vi "Main.vi"() -> ()   [LabVIEW 2024]
doc: "This Continuous Measurement sample project is based on the Queued Message Handler template.\n\nThe Event Handling Loop generates messages based on user interface actions.\n\nThe Message Handling Loop processes messages generated by the Event Handling Loop, or by other messages. There are also Acquisition and Logging message handling loop subVIs, and a chart updating loop."
uses:
  Acquisition/Acquisition.lvlib
  Logging/Logging.lvlib
  support/User Event - Stop/User Event - Stop.lvlib
  controls/UI Data.ctl
  support/Message Queue/Message Queue.lvlib
  support/Message Queue/Enqueue Message (Single).vi
  <vilib>/ErrorRing/Error Ring.xnode
  controls/UI State.ctl
  <vilib>/Utility/error.llb/Error Cluster From Error Code.vi
  controls/channelDefinition.ctl
  controls/self.ctl
  controls/dataRefs.ctl
panel:
  out "Data":dbl[][](graph)
  in  "Force Trigger":bool
  in  "Start":bool
  in  "Stop":bool
  out "Status":string
  in  "Exit":bool
  # "Continuous Measurement and Logging (NI-DAQmx)"
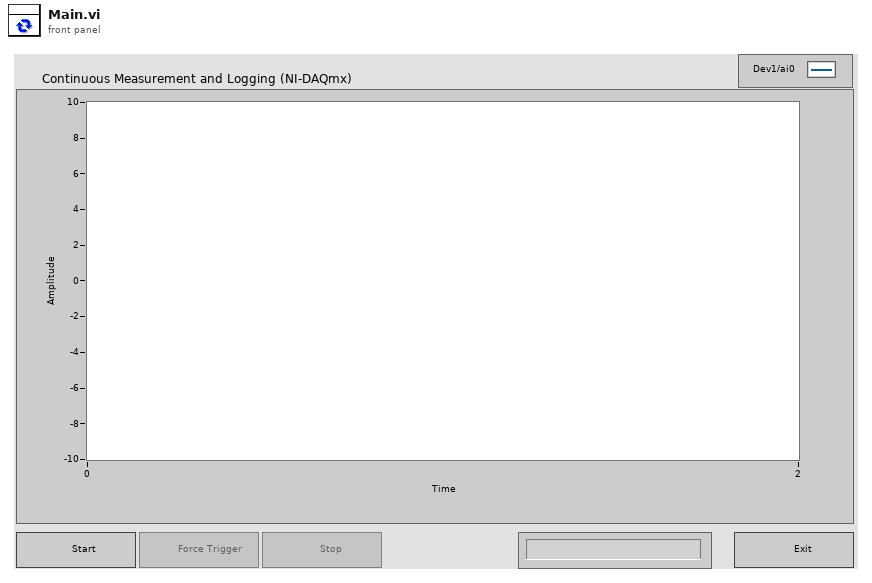
[diagram p1: front panel]
types:
  T1 = typedef "dataRefs.ctl" = cluster{"dataTypeConstant":cluster{"data":dbl[][], "refDes":string[]}, "user_I":refnum<notifier>, "user_O":refnum<notifier>, "daq_O":refnum<notifier>, "logging":refnum<queue>, "daq_I":refnum<queue>}
  T2 = typedef "self.ctl" = cluster{"refDes":string, "IP":string, "DI":i32, "DO":i32, "AI":i32, "AO":i32, "Description":string, "TC":i32, "channelDefinitions":T3[]}
  T3 = typedef "channelDefinition.ctl" = cluster{"channel":string, "refDes":string, "units":string, "slope":dbl, "offset":dbl, "type":string}
  T4 = typedef "UI State.ctl" = enum16{"Idle", "Acquiring and Logging", "Waiting for Exit", "Waiting for Exit (Acq Stopped)", "Waiting for Exit (Log Stopped)", "Waiting for Stop", "Waiting for Stop (Acq Stopped)", "Waiting for Stop (Log Stopped)"}
  T5 = typedef "UI Data.ctl" = cluster{"Start Ref":refnum<vi>, "Trigger Ref":refnum<vi>, "Stop Ref":refnum<vi>, "Settings Ref":refnum<vi>, "Status Ref":refnum<vi>, "Exit Ref":refnum<vi>, "Data Ref":refnum<vi>}
  T6 = typedef "Message Queue.lvlib/All Message Queues.ctl" = cluster{"UI":refnum<queue>, "Acquisition":refnum<queue>, "Logging":refnum<queue>}
  T7 = enum8{"Enabled", "Disabled", "Disabled and Grayed Out"}
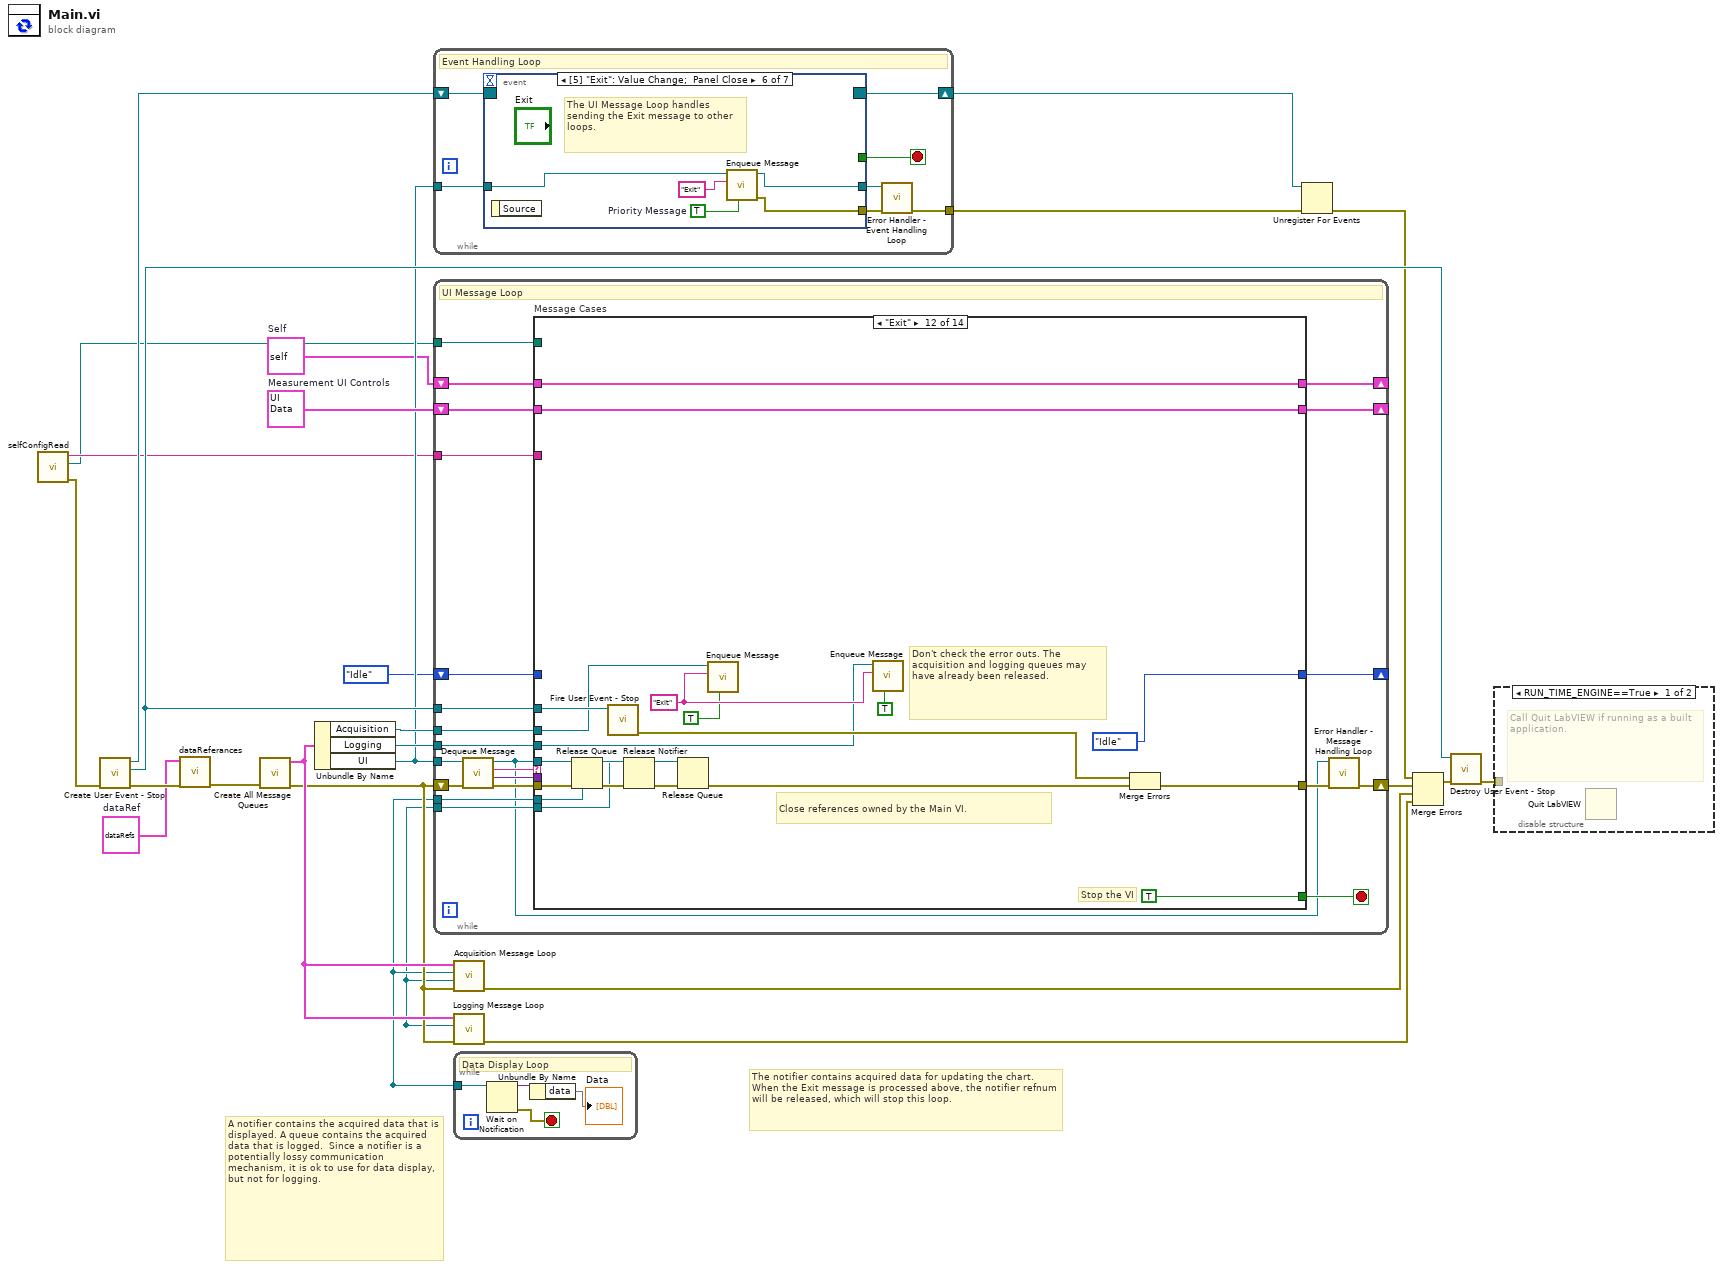
[diagram p0: block diagram]
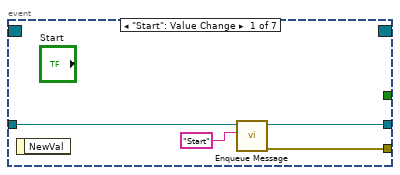
[diagram p3: hidden frame]
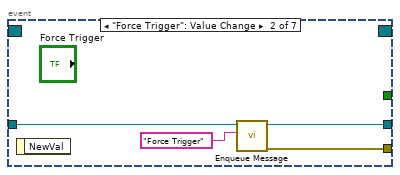
[diagram p4: hidden frame]
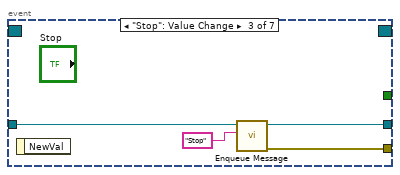
[diagram p5: hidden frame]
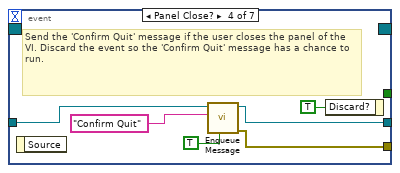
[diagram p6: hidden frame]
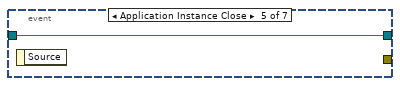
[diagram p7: hidden frame]
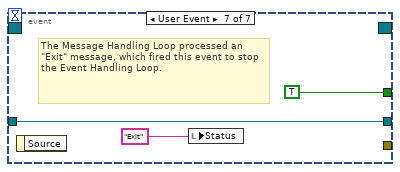
[diagram p8: hidden frame]
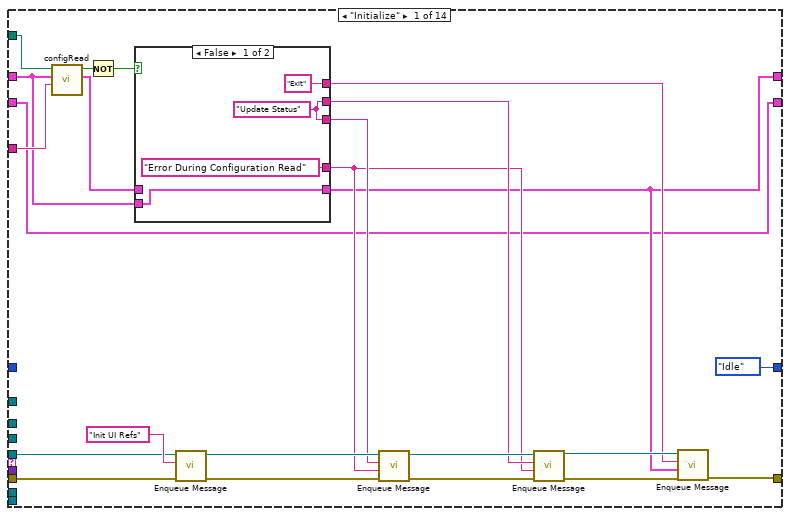
[diagram p9: hidden frame]
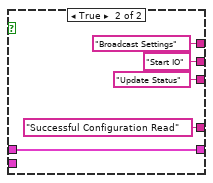
[diagram p10: hidden frame]
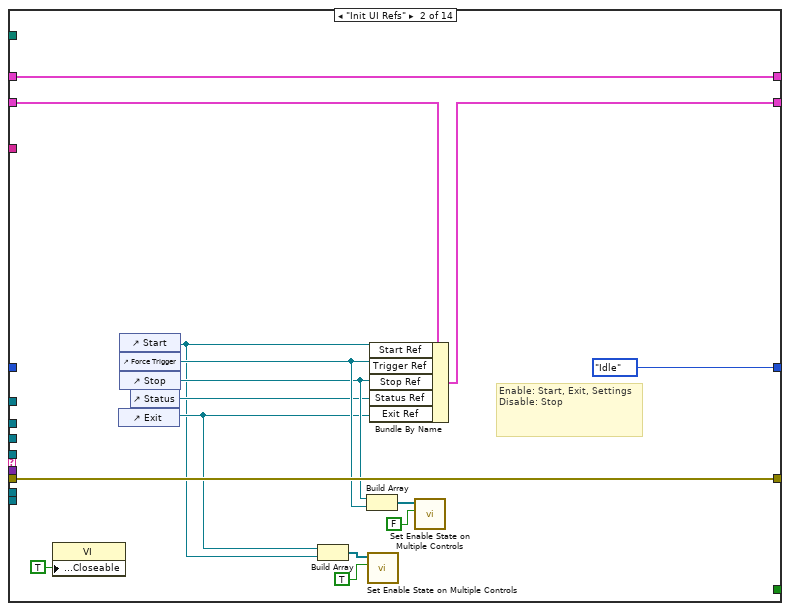
[diagram p11: hidden frame]
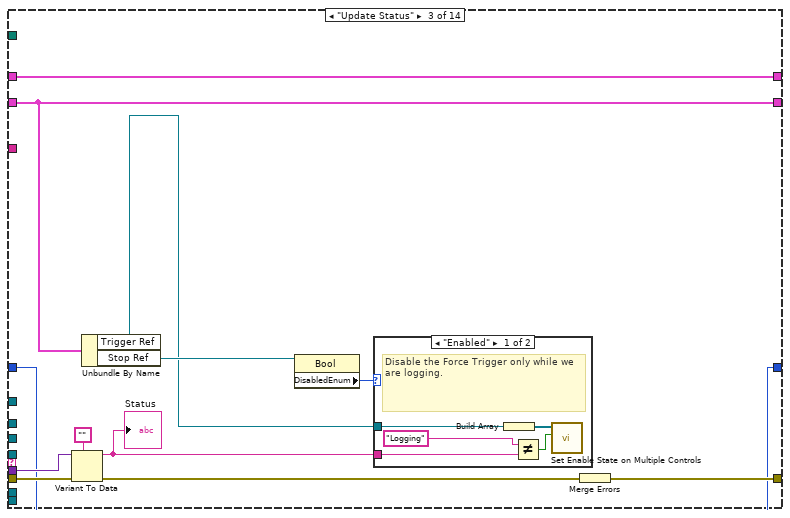
[diagram p12: hidden frame]
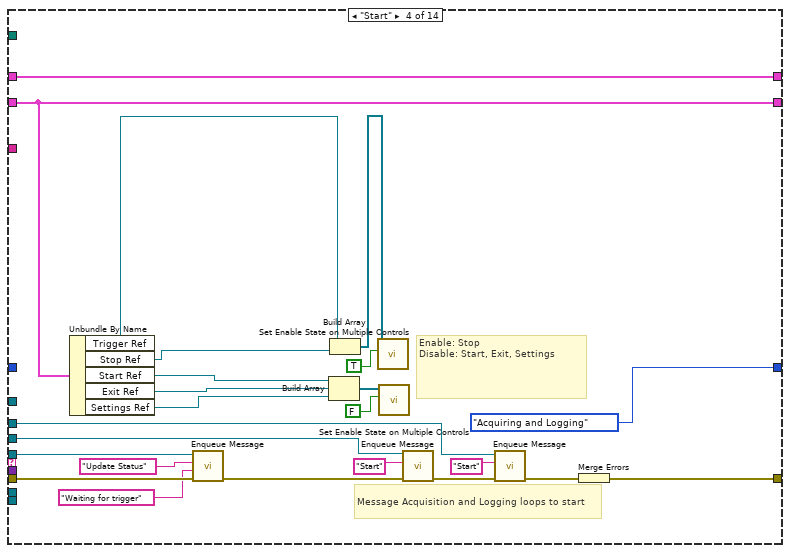
[diagram p14: hidden frame]
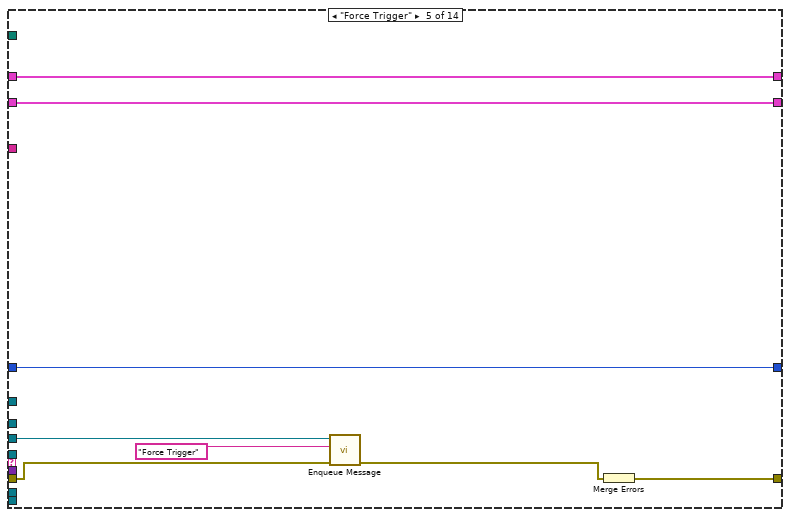
[diagram p15: hidden frame]
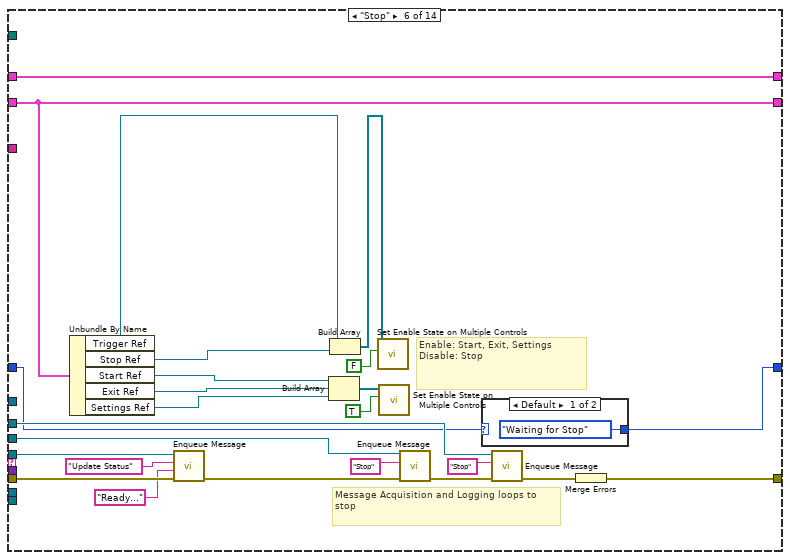
[diagram p16: hidden frame]
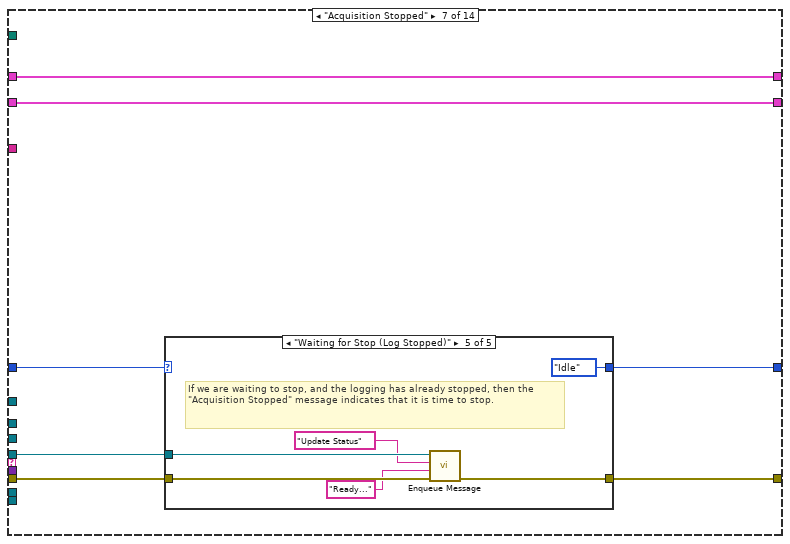
[diagram p18: hidden frame]
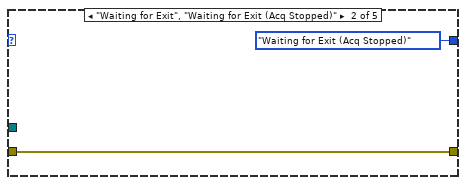
[diagram p20: hidden frame]
diagram:
  w1 = T1 {"dataTypeConstant"={"data"=[], "refDes"=[]}, "user_I"=refnum, "user_O"=refnum, "daq_O"=refnum, "logging"=refnum, "daq_I"=refnum}  # dataRef
  w9 = T2 {"refDes"="ERR000", "IP"="localhost", "DI"=0, "DO"=0, "AI"=0, "AO"=0, "Description"="ERR", "TC"=0, "channelDefinitions"=[]}  # Self
  w15 = T5 {"Start Ref"=refnum, "Trigger Ref"=refnum, "Stop Ref"=refnum, "Settings Ref"=refnum, "Status Ref"=refnum, "Exit Ref"=refnum, "Data Ref"=refnum}  # Measurement UI Controls
  # "A notifier contains the acquired data that is displayed. A queue contains the acquired data that is logged.  Since a notifier is a potentially lossy communication mechanism, it is ok to use for data display, but not for logging."
  # "The notifier contains acquired data for updating the chart. When the Exit message is processed above, the notifier refnum will be released, which will stop this loop."
  n1 = call "selfConfigRead.vi"() -> ("error out"=w7:errorcluster, "configPath"=w6:path, "refDes"=w8:string)  [unwired: 9 in]
  n2 = call "Create User Event - Stop.vi"("error in (no error)"=w7) -> ("error out"=w3:errorcluster, "User Event - Stop"=w22:refnum<user-event>, "Stop Event Registration Refnum"=w23:refnum<event-registration>)  [unwired: 8 in]
  n3 = call "dataReferances.vi"("error in (no error)"=w3, "dataRefIn"=w1) -> ("error out"=w2:errorcluster)  [unwired: 8 in, 1 out]
  n4 = call "Create All Message Queues.vi"("error in (no error)"=w2) -> ("error out"=w18:errorcluster, "Message Queues out"=w20:T6)  [unwired: 9 in]
  n5 = Unbundle By Name(w20) -> ("Acquisition"=w14:refnum<queue>, "Logging"=w13:refnum<queue>, "UI"=w12:refnum<queue>)
  n6 = while {
    tunnel: w12 -> [w32]
    tunnel: [w27] -> w25
    shift-right: [w31] -> w16
    shift-left: w23 -> [w33]
    stop <- w30 stop-if-true
    # "Event Handling Loop"
    n7 = event shown="[5] \"Exit\": Value Change;  Panel Close" {
      selector: w33 -> [_ _ _ _ _ _ _]
      dyn-events: [_ _ _ _ _ _ _] -> w31
      timeout: _ -> [_ _ _ _ _ _ _]
      tunnel: [_ _ _ _ _ _ TRUE ("Discard?")] -> w30
      tunnel: w32 -> [w35 w40 w44 w51 w52 w54 w58]
      tunnel: [w37 w39 w43 w46 _ w57 _] -> w28
      tunnel: [w34 w38 w42 w47 w52 w53 w58] -> w29
      event "Start": Value Change {
        n8 = event-data() -> ()  [unwired: 1 in, 1 out]
        n9 = call-poly "Enqueue Message.vi"("Message"="Start", "Message Queue"=w35) -> ("error out"=w37:errorcluster, "dup Message Queue"=w34:refnum<queue>)  [unwired: 8 in]
      }
      event "Force Trigger": Value Change {
        n10 = event-data() -> ()  [unwired: 1 in, 1 out]
        n11 = call-poly "Enqueue Message.vi"("Message"="Force Trigger", "Message Queue"=w40) -> ("error out"=w39:errorcluster, "dup Message Queue"=w38:refnum<queue>)  [unwired: 8 in]
      }
      event "Stop": Value Change {
        n12 = event-data() -> ()  [unwired: 1 in, 1 out]
        n13 = call-poly "Enqueue Message.vi"("Message"="Stop", "Message Queue"=w44) -> ("error out"=w43:errorcluster, "dup Message Queue"=w42:refnum<queue>)  [unwired: 8 in]
      }
      event Panel Close? {
        # "Send the 'Confirm Quit' message if the user closes the panel of the VI. Discard the event so the 'Confirm Quit' message has a chance to run."
        n14 = event-data() -> ()  [unwired: 1 in, 1 out]
        n15 = call-poly "Enqueue Message.vi"("Priority Message? (F)"=TRUE, "Message"="Confirm Quit", "Message Queue"=w51) -> ("error out"=w46:errorcluster, "dup Message Queue"=w47:refnum<queue>)  [unwired: 7 in]
        n16 = event-data("Discard?"=TRUE) -> ()  [unwired: 1 in, 1 out]
      }
      event Application Instance Close {
        n17 = event-data() -> ()  [unwired: 1 in, 1 out]
      }
      event "Exit": Value Change; Panel Close {
        w55 = TRUE  # Priority Message
        # "The UI Message Loop handles sending the Exit message to other loops."
        n18 = event-data() -> ()  [unwired: 1 in, 1 out]
        n19 = call-poly "Enqueue Message.vi"("Priority Message? (F)"=w55, "Message"="Exit", "Message Queue"=w54) -> ("error out"=w57:errorcluster, "dup Message Queue"=w53:refnum<queue>)  [unwired: 7 in]
      }
      event User Event {
        # "The Message Handling Loop processed an \"Exit\" message, which fired this event to stop the Event Handling Loop."
        n20 = event-data() -> ()  [unwired: 1 in, 1 out]
        n21 = local write "Status"("Exit" ("Exit String")) -> ()
      }
    }
    n22 = call "Error Handler - Event Handling Loop.vi"("error in (no error)"=w28, "Message Queue"=w29) -> ("dup error in"=w27:errorcluster)  [unwired: 8 in, 1 out]
  }
  n23 = Unregister For Events(event registration refnum=w16, error in=w25) -> (error out=w17:errorcluster)
  n24 = while {
    tunnel: w12 -> [w76]
    tunnel: w22 -> [w81]
    shift-right: [w66] -> w26
    shift-left: w18 -> [w80]
    shift-right: [w75] -> _
    shift-left: w9 -> [w74]
    shift-right: [w72] -> _
    shift-left: w15 -> [w73]
    tunnel: w14 -> [w71]
    tunnel: w13 -> [w70]
    tunnel: [w69] -> w5
    tunnel: w4 -> [w68]
    shift-right: [w63] -> _
    shift-left: UI_State."Idle" ("UI State") -> [w64]
    tunnel: w6 -> [w62]
    tunnel: w8 -> [w61]
    stop <- w82 stop-if-true
    # "UI Message Loop"
    n25 = call "Dequeue Message.vi"("error in (no error)"=w80, "Message Queue"=w76) -> ("error out"=w79:errorcluster, "Message Data"=w77:variant, "Message"=w78:string, "dup Message Queue"=w65:refnum<queue>)  [unwired: 6 in]
    n26 = case "Message Cases" shown="\"Exit\"" w78 {
      selector: w78 -> [_ _ _ _ _ _ _ _ _ _ _ _ _ w332]
      tunnel: w65 -> [w104 _ _ w169 _ w202 w206 w231 _ w272 w282 w315 _ _]
      tunnel: w79 -> [w103 w129 w140 w168 w175 w201 w208 w233 w262 w276 w281 w323 w330 _]
      tunnel: [w98 w129 w141 w170 w178 w203 w207 w232 w265 w267 w280 w324 w329 w333] -> w67
      tunnel: [_ _ _ _ _ _ _ _ _ _ _ TRUE _ _] -> w82
      tunnel: w77 -> [_ _ w139 _ _ _ _ _ _ w275 _ _ _ _]
      tunnel: w81 -> [_ _ _ _ _ _ _ _ _ _ _ w322 _ _]
      tunnel: [w84 w128 w136 w167 w177 w200 w212 w237 w256 w278 w285 w320 w328 w335] -> w75
      tunnel: w74 -> [w95 w128 w136 w167 w177 w200 w212 w237 w256 w278 w285 w320 w328 w335]
      tunnel: w73 -> [w83 w127 w135 w164 w176 w197 w211 w236 w260 w277 w284 w318 w327 w334]
      tunnel: [w83 w126 w135 w164 w176 w197 w211 w236 w260 w277 w284 w318 w327 w334] -> w72
      tunnel: w71 -> [_ _ _ w151 _ w184 _ _ w259 _ _ w317 _ _]
      tunnel: w70 -> [_ _ _ w154 w172 w187 _ _ w258 _ _ w316 _ _]
      tunnel: w69 -> [_ _ _ _ _ _ _ _ _ _ _ w314 _ _]
      tunnel: w68 -> [_ _ _ _ _ _ _ _ _ _ _ w310 _ _]
      tunnel: w64 -> [_ _ w130 _ w171 w180 w210 w235 w257 w266 w283 _ w326 w331]
      tunnel: [UI_State."Idle" ("UI State") UI_State."Idle" ("UI State") w130 UI_State."Acquiring and Logging" ("UI State") w171 w179 w209 w234 w257 w266 w279 UI_State."Idle" ("UI State") w326 w331] -> w63
      tunnel: w62 -> [w100 _ _ _ _ _ _ _ _ _ _ _ _ _]
      tunnel: w61 -> [w99 _ _ _ _ _ _ _ _ _ _ _ _ _]
      frame "Initialize" {
        # "Initialize - Get configuration settings, then message the UI to initialize, and broadcast the settings to the other message loops."
        n27 = call "configRead.vi"("refDes"=w99, "Self"=w95, "configPath"=w100) -> ("Self"=w96:T2, "Cancel/Err"=w101:bool)  [unwired: 7 in]
        n28 = Not(x=w101) -> (.not. x?=w97:bool)
        n29 = case shown="False" w97 {
          tunnel: w96 -> [_ w114]
          tunnel: [w109 w114] -> w84
          tunnel: w95 -> [w109 _]
          tunnel: ["Exit" ("Message") "Broadcast Settings" ("Message")] -> w86
          tunnel: [w106 "Start IO" ("Message")] -> w87
          tunnel: [w106 "Update Status" ("Message")] -> w88
          tunnel: ["Error During Configuration Read" "Successful Configuration Read"] -> w85
          frame False {
            w106 = "Update Status" ("Message")
          }
          frame True {
          }
        }
        n30 = call-poly "Enqueue Message.vi"("error in (no error)"=w103, "Message"="Init UI Refs", "Message Queue"=w104) -> ("error out"=w93:errorcluster, "dup Message Queue"=w94:refnum<queue>)  [unwired: 7 in]
        n31 = call-poly "Enqueue Message.vi"("error in (no error)"=w93, "Message Data"=w85, "Message"=w88, "Message Queue"=w94) -> ("error out"=w91:errorcluster, "dup Message Queue"=w92:refnum<queue>)  [unwired: 6 in]
        n32 = call-poly "Enqueue Message.vi"("error in (no error)"=w91, "Message Data"=w85, "Message"=w87, "Message Queue"=w92) -> ("error out"=w90:errorcluster, "dup Message Queue"=w89:refnum<queue>)  [unwired: 6 in]
        n33 = call-poly "Enqueue Message.vi"("error in (no error)"=w90, "Message Data"=w84, "Message"=w86, "Message Queue"=w89) -> ("error out"=w98:errorcluster)  [unwired: 6 in, 1 out]
      }
      frame "Init UI Refs" {
        # "Enable: Start, Exit, Settings\nDisable: Stop"
        # "Init UI Refs - Store control references for UI controls.  Also enable/disable controls appropriately."
        n34 = property class="VI"("Front Panel.Closeable"=TRUE ("Front Panel Window:Closeable")) -> ()  [unwired: 2 in, 2 out]
        n35 = control-ref of="Exit"() -> (w116:refnum<vi>)
        n36 = control-ref of="Start"() -> (w115:refnum<vi>)
        n37 = control-ref of="Force Trigger"() -> (w121:refnum<vi>)
        n38 = control-ref of="Stop"() -> (w120:refnum<vi>)
        n39 = control-ref of="Status"() -> (w117:refnum<vi>)
        n40 = Build Array(w116, w115) -> (w123:refnum<vi>[])
        n41 = Build Array(w120, w121) -> (w119:refnum<vi>[])
        n42 = call "Set Enable State on Multiple Controls.vi"("Enable?"=TRUE, "Controls"=w123) -> ()  [unwired: 10 in]
        n43 = Bundle By Name(cluster=w127, "Start Ref"=w115, "Trigger Ref"=w121, "Stop Ref"=w120, "Status Ref"=w117, "Exit Ref"=w116) -> (w126:T5)
        n44 = call "Set Enable State on Multiple Controls.vi"("Enable?"=FALSE, "Controls"=w119) -> ()  [unwired: 10 in]
      }
      frame "Update Status" {
        # "Update Display - Convert the message data to a string to display in the Status indicator."
        n45 = Variant To Data(error in=w140, type="", Variant=w139) -> (data=w132:string, error out=w137:errorcluster)
        "Status" <- w132
        n46 = Unbundle By Name(w135) -> ("Trigger Ref"=w131:refnum<vi>, "Stop Ref"=w134:refnum<vi>)
        n47 = property class="Bool"(reference=w134) -> ("DisabledEnum"=w133:T7)  [unwired: 1 in, 2 out]
        n48 = case shown="\"Enabled\"" w133 {
          tunnel: w132 -> [w144 _]
          tunnel: w131 -> [w145 _]
          frame "Enabled" {
            # "Disable the Force Trigger only while we are logging."
            n49 = Build Array(w145) -> (w146:refnum<vi>[])
            n50 = Not Equal?(x="Logging" ("Logging"), y=w144) -> (x != y?=w142:bool)
            n51 = call "Set Enable State on Multiple Controls.vi"("Enable?"=w142, "Controls"=w146) -> ()  [unwired: 10 in]
          }
          frame "Disabled", Default {
          }
        }
        n52 = Merge Errors(w137) -> (w141:errorcluster)
      }
      frame "Start" {
        # "Message Acquisition and Logging loops to start"
        # "Enable: Stop\nDisable: Start, Exit, Settings"
        # "Start - Enable/Disable buttons appropriately for an acquisition that has started, and update status display."
        n53 = Unbundle By Name(w164) -> ("Trigger Ref"=w148:refnum<vi>, "Stop Ref"=w149:refnum<vi>, "Start Ref"=w159:refnum<vi>, "Exit Ref"=w158:refnum<vi>, "Settings Ref"=w157:refnum<vi>)
        n54 = call-poly "Enqueue Message.vi"("error in (no error)"=w168, "Message Data"="Waiting for trigger" ("Waiting for trigger"), "Message"="Update Status", "Message Queue"=w169) -> ("error out"=w156:errorcluster)  [unwired: 6 in, 1 out]
        n55 = Build Array(w159, w158, w157) -> (w162:refnum<vi>[])
        n56 = Build Array(w148, w149) -> (w161:refnum<vi>[])
        n57 = call "Set Enable State on Multiple Controls.vi"("Enable?"=TRUE, "Controls"=w161) -> ()  [unwired: 10 in]
        n58 = call "Set Enable State on Multiple Controls.vi"("Enable?"=FALSE, "Controls"=w162) -> ()  [unwired: 10 in]
        n59 = call-poly "Enqueue Message.vi"("error in (no error)"=w156, "Message"="Start", "Message Queue"=w154) -> ("error out"=w153:errorcluster)  [unwired: 7 in, 1 out]
        n60 = call-poly "Enqueue Message.vi"("error in (no error)"=w153, "Message"="Start", "Message Queue"=w151) -> ("error out"=w152:errorcluster)  [unwired: 7 in, 1 out]
        n61 = Merge Errors(w152) -> (w170:errorcluster)
      }
      frame "Force Trigger" {
        # "Force Trigger - send a message to the Logging message loop to start logging."
        n62 = call-poly "Enqueue Message.vi"("error in (no error)"=w175, "Message"="Force Trigger", "Message Queue"=w172) -> ("error out"=w174:errorcluster)  [unwired: 7 in, 1 out]
        n63 = Merge Errors(w174) -> (w178:errorcluster)
      }
      frame "Stop" {
        # "Message Acquisition and Logging loops to stop"
        # "Enable: Start, Exit, Settings\nDisable: Stop"
        # "Stop - Enable/Disable buttons appropriately for an acquisition that has stopped, and update status display."
        n64 = Unbundle By Name(w197) -> ("Trigger Ref"=w181:refnum<vi>, "Stop Ref"=w182:refnum<vi>, "Start Ref"=w192:refnum<vi>, "Exit Ref"=w191:refnum<vi>, "Settings Ref"=w190:refnum<vi>)
        n65 = call-poly "Enqueue Message.vi"("error in (no error)"=w201, "Message Data"="Ready..." ("Ready..."), "Message"="Update Status", "Message Queue"=w202) -> ("error out"=w189:errorcluster)  [unwired: 6 in, 1 out]
        n66 = Build Array(w192, w191, w190) -> (w195:refnum<vi>[])
        n67 = Build Array(w181, w182) -> (w194:refnum<vi>[])
        n68 = call "Set Enable State on Multiple Controls.vi"("Enable?"=FALSE, "Controls"=w194) -> ()  [unwired: 10 in]
        n69 = call "Set Enable State on Multiple Controls.vi"("Enable?"=TRUE, "Controls"=w195) -> ()  [unwired: 10 in]
        n70 = call-poly "Enqueue Message.vi"("error in (no error)"=w189, "Message"="Stop", "Message Queue"=w187) -> ("error out"=w186:errorcluster)  [unwired: 7 in, 1 out]
        n71 = case shown="Default" w180 {
          selector: w180 -> [_ w205]
          tunnel: [UI_State."Waiting for Stop" ("UI State") w205] -> w179
          frame Default {
          }
          frame "Waiting for Exit" {
          }
        }
        n72 = call-poly "Enqueue Message.vi"("error in (no error)"=w186, "Message"="Stop", "Message Queue"=w184) -> ("error out"=w185:errorcluster)  [unwired: 7 in, 1 out]
        n73 = Merge Errors(w185) -> (w203:errorcluster)
      }
      frame "Acquisition Stopped" {
        # "Logic for determining what action to take when the acquisition has stopped."
        n74 = case shown="\"Waiting for Stop (Log Stopped)\"" w210 {
          selector: w210 -> [w214 _ _ _ _]
          tunnel: [w214 UI_State."Waiting for Exit (Acq Stopped)" ("UI State") UI_State."Waiting for Stop (Acq Stopped)" ("UI State") UI_State."Idle" ("UI State") UI_State."Idle" ("UI State")] -> w209
          tunnel: w208 -> [w213 w215 w217 w223 w229]
          tunnel: [w213 w215 w217 w222 w228] -> w207
          tunnel: w206 -> [_ _ _ w221 w227]
          frame Default {
          }
          frame "Waiting for Exit", "Waiting for Exit (Acq Stopped)" {
          }
          frame "Waiting for Stop", "Waiting for Stop (Acq Stopped)" {
          }
          frame "Waiting for Exit (Log Stopped)" {
            # "If we are waiting to exit, and the logging has already stopped, then the \"Acquisition Stopped\" message indicates that it is time to exit."
            n75 = call-poly "Enqueue Message.vi"("Priority Message? (F)"=TRUE, "error in (no error)"=w223, "Message"="Exit", "Message Queue"=w221) -> ("error out"=w222:errorcluster)  [unwired: 6 in, 1 out]
          }
          frame "Waiting for Stop (Log Stopped)" {
            # "If we are waiting to stop, and the logging has already stopped, then the \"Acquisition Stopped\" message indicates that it is time to stop."
            n76 = call-poly "Enqueue Message.vi"("error in (no error)"=w229, "Message Data"="Ready..." ("Message"), "Message"="Update Status", "Message Queue"=w227) -> ("error out"=w228:errorcluster)  [unwired: 6 in, 1 out]
          }
        }
      }
      frame "Logging Stopped" {
        # "Logic for determining what action to take when the logging has stopped."
        n77 = case shown="\"Waiting for Stop (Acq Stopped)\"" w235 {
          selector: w235 -> [w239 _ _ _ _]
          tunnel: [w239 UI_State."Waiting for Exit (Log Stopped)" ("UI State") UI_State."Waiting for Stop (Log Stopped)" ("UI State") UI_State."Idle" ("UI State") UI_State."Idle" ("UI State")] -> w234
          tunnel: w233 -> [w238 w240 w242 w248 w254]
          tunnel: [w238 w240 w242 w247 w253] -> w232
          tunnel: w231 -> [_ _ _ w246 w252]
          frame Default {
          }
          frame "Waiting for Exit", "Waiting for Exit (Log Stopped)" {
          }
          frame "Waiting for Stop", "Waiting for Stop (Log Stopped)" {
          }
          frame "Waiting for Exit (Acq Stopped)" {
            # "If we are waiting to exit, and the acquisition has already stopped, then the \"Logging Stopped\" message indicates that it is time to exit."
            n78 = call-poly "Enqueue Message.vi"("Priority Message? (F)"=TRUE, "error in (no error)"=w248, "Message"="Exit", "Message Queue"=w246) -> ("error out"=w247:errorcluster)  [unwired: 6 in, 1 out]
          }
          frame "Waiting for Stop (Acq Stopped)" {
            # "If we are waiting to stop, and the acquisition has already stopped, then the \"Logging Stopped\" message indicates that it is time to stop."
            n79 = call-poly "Enqueue Message.vi"("error in (no error)"=w254, "Message Data"="Ready..." ("Message"), "Message"="Update Status", "Message Queue"=w252) -> ("error out"=w253:errorcluster)  [unwired: 6 in, 1 out]
          }
        }
      }
      frame "Broadcast settings" {
        w261 = "Update Settings" ("Message")
        # "Send the 'Update Settings' message to the Logging and Acquisition message loops."
        n80 = call-poly "Enqueue Message.vi"("Message Data"=w256, "Message"=w261, "Message Queue"=w259) -> ("error out"=w264:errorcluster)  [unwired: 7 in, 1 out]
        n81 = call-poly "Enqueue Message.vi"("error in (no error)"=w264, "Message Data"=w256, "Message"=w261, "Message Queue"=w258) -> ("error out"=w263:errorcluster)  [unwired: 6 in, 1 out]
        n82 = Merge Errors(w263, w262) -> (w265:errorcluster)
      }
      frame "Error" {
        # "Error - Check the error message data and respond accordingly. This message is sent by the \"Error Handler\" VIs at the end of each loop in this application."
        n83 = Variant To Data(error in=w276, type=errorcluster {"status"=FALSE, "code"=0, "source"=""} ("error out"), Variant=w275) -> (data=w273:errorcluster, error out=w269:errorcluster)
        n84 = call <vilib>:"Simple Error Handler.vi"("error in (no error)"=w273) -> ()  [unwired: 4 in, 5 out]
        n85 = call-poly "Enqueue Message.vi"("Priority Message? (F)"=TRUE, "Message"="Exit", "Message Queue"=w272) -> ("error out"=w268:errorcluster)  [unwired: 7 in, 1 out]
        n86 = Merge Errors(w268, w269) -> (w267:errorcluster)
      }
      frame "Confirm Quit" {
        # "Confirm Quit - Message that can confirm whether or not the user wants to exit the application."
        n87 = case shown="\"Acquiring and Logging\"" w283 {
          tunnel: w282 -> [w290 w296]
          tunnel: w281 -> [w289 w294]
          tunnel: [w286 w293] -> w280
          tunnel: [UI_State."Idle" ("UI State") w292] -> w279
          frame Default {
            # "If 'Confirm Quit' comes in while the system is idle, there is no need for a confirmation message."
            n88 = call-poly "Enqueue Message.vi"("Priority Message? (F)"=TRUE, "error in (no error)"=w289, "Message"="Exit", "Message Queue"=w290) -> ("error out"=w286:errorcluster)  [unwired: 6 in, 1 out]
          }
          frame "Acquiring and Logging" {
            n89 = Two Button Dialog(message="Are you sure you want to quit while the acquisition is running?" ("Confirm Quit Message"), 1:"No" ("No"), 2:"Yes" ("Yes")) -> (T button?=w295:bool)
            n90 = case shown="True" w295 {
              tunnel: w296 -> [_ w306]
              tunnel: w294 -> [w300 w305]
              tunnel: [w300 w304] -> w293
              tunnel: [UI_State."Acquiring and Logging" ("UI State") UI_State."Waiting for Exit" ("UI State")] -> w292
              frame False {
                # "User did not want to quit."
              }
              frame True {
                n91 = call-poly "Enqueue Message.vi"("error in (no error)"=w305, "Message"="Stop", "Message Queue"=w306) -> ("error out"=w304:errorcluster)  [unwired: 7 in, 1 out]
              }
            }
          }
        }
      }
      frame "Exit" {
        w319 = "Exit" ("Message")
        # "Don't check the error outs. The acquisition and logging queues may have already been released."
        # "Close references owned by the Main VI."
        # "Stop the VI"
        # "Exit - Fire the User Event to stop the Event Handling Loop.  Also send Exit messages to the Acquisition and Logging loops."
        n92 = Release Queue(queue=w315, error in (no error)=w323) -> (error out=w313:errorcluster)  [unwired: 1 in, 2 out]
        n93 = call "Fire User Event - Stop.vi"("User Event - Stop"=w322) -> ("error out"=w321:errorcluster)  [unwired: 10 in]
        n94 = Release Notifier(notifier=w314, error in (no error)=w313) -> (error out=w312:errorcluster)  [unwired: 1 in, 2 out]
        n95 = Release Queue(queue=w310, error in (no error)=w312) -> (error out=w311:errorcluster)  [unwired: 1 in, 2 out]
        n96 = call-poly "Enqueue Message.vi"("Priority Message? (F)"=TRUE, "Message"=w319, "Message Queue"=w317) -> ()  [unwired: 7 in, 2 out]
        n97 = call-poly "Enqueue Message.vi"("Priority Message? (F)"=TRUE, "Message"=w319, "Message Queue"=w316) -> ()  [unwired: 7 in, 2 out]
        n98 = Merge Errors(w321, w311) -> (w324:errorcluster)
      }
      frame "---Copy This Frame---" {
        # "Duplicate this frame when creating new messages.  Change this comment in the duplicated frame to describe this message."
        n99 = Merge Errors(w330) -> (w329:errorcluster)
      }
      frame Default {
        # "'Default' case only runs if there is a message that isn't defined in any of the other cases.  Output a programming error."
        n100 = xnode "Error Ring"("parameter 0"=w332) -> ("error out"=w333:errorcluster)
      }
    }
    n101 = call "Error Handler - Message Handling Loop.vi"("error in (no error)"=w67, "Message Queue"=w65) -> ("dup error in"=w66:errorcluster)  [unwired: 8 in, 1 out]
  }
  n102 = call "Acquisition Message Loop.vi"("error in (no error)"=w18, "Data Notifier"=w5, "Message Queues"=w20) -> ("error out"=w21:errorcluster, "Data Queue"=w4:refnum<queue>)  [unwired: 7 in]
  n103 = call "Logging Message Loop.vi"("error in (no error)"=w18, "Data Queue"=w4, "Message Queues"=w20) -> ("error out"=w19:errorcluster)  [unwired: 8 in]
  n104 = while "Data Display Loop" {
    tunnel: w5 -> [w346]
    stop <- w345 stop-if-true
    # "Data Display Loop"
    n105 = Wait on Notification(notifier=w346) -> (notification=w344:variant, error out=w345:errorcluster)  [unwired: 3 in, 2 out]
    n106 = Unbundle By Name(w344) -> ("data"=→"Data")
  }
  n107 = Merge Errors(w17, w26, w21, w19) -> (w24:errorcluster)
  n108 = call "Destroy User Event - Stop.vi"("error in (no error)"=w24, "User Event - Stop"=w22) -> ("error out"=w11:errorcluster)  [unwired: 9 in]
  n109 = disable-structure shown="RUN_TIME_ENGINE==True" {
    disable-tunnel: w11 -> [_ _]
    frame condition #0 {
      # "Call Quit LabVIEW if running as a built application."
      n110 = Quit LabVIEW() -> ()  [unwired: 1 in]
    }
    frame condition #1 (active) {
    }
  }
